vi "openFile.vi"(8 "error in (no error)":errorcluster, 11 "Handler.File.Text in":refnum<class "Handler.File.Text.lvclass">) -> (0 "error out":errorcluster, 3 "Handler.File.Text out":refnum<class "Handler.File.Text.lvclass">)   [LabVIEW 2017, in "Error Log.lvlib" / "Handler.File.Text.lvclass"]
uses:
  Handler.File.Text.lvclass
  \\192.168.1.40\Neosoft/Partage/Dossiers Personnels/BRO/DevTools_BR/wc/ErrorLog/src/Handler.File/Handler.File.lvclass
  Handler.File/Handler.File.lvclass/Handler.File.ctl
  Handler.File.Text.lvclass/Handler.File.Text.ctl
  Handler.File/Get File Path.vi
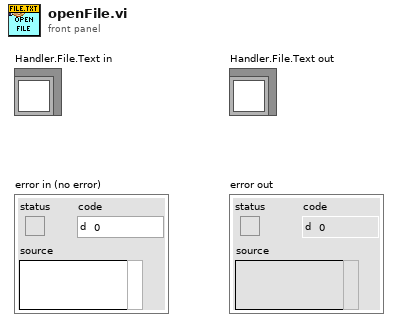
[diagram p1: front panel]
types:
  T1 = enum16{"open", "replace", "create", "open or create", "replace or create", "replace or create with confirmation"}
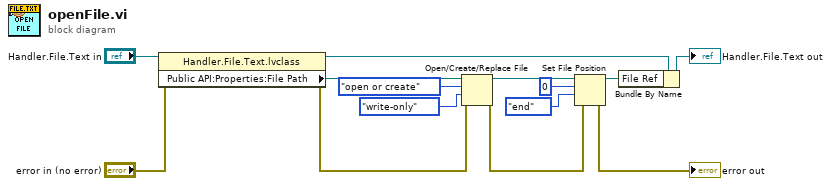
[diagram p0: block diagram]
diagram:
  n1 = property class="Handler.File.Text.lvclass"(reference="Handler.File.Text in", error in="error in (no error)") -> (reference out=w13:refnum<class "Handler.File.Text.lvclass">, error out=w4:errorcluster, "Public API:Properties:File Path"=w5:path)
  n2 = Open/Create/Replace File(file path (use dialog)=w5, error in=w4, operation (0:open)=T1."open or create", access (0:read/write)=enum16{"read/write", "read-only", "write-only"}."write-only") -> (refnum out=w9:refnum<file>, error out=w10:errorcluster)  [unwired: 2 in, 1 out]
  n3 = Set File Position(offset (in bytes) (0)=i64 0, refnum=w9, from (0:start)=enum16{"start", "end", "current"}."end", error in=w10) -> (refnum out=w1:refnum<file>, error out=→"error out":errorcluster)
  n4 = Bundle By Name(cluster=w13, "File Ref"=w1) -> (→"Handler.File.Text out":refnum<class "Handler.File.Text.lvclass">)
